vi "MainImage.vi"() -> ()   [LabVIEW 2019]
panel:
  in  "stop":bool
  in  "Tab Control":enum32{"Pressure", "Temperature", "Image"}(tab)
  out "Waveform Chart 2":cluster{dbl, dbl, dbl}(graph)
  in  "VISA resource name":refnum<visa-resource-name>="COM3"
  in  "termination char\n(0xA = '\\n' = LF)":u8=13 format="%.0x"
  in  "Recieve Data":bool
  out "Waveform Chart":T1(graph)
  in  "physical channels":tag="PXI1Slot2/ai2"
  in  "resistance configuration":i32(ring)=2 items=["2-Wire"=2, "3-Wire"=3, "4-Wire"=4]
  in  "valor":i32
  out "Gauge 1":dbl
  out "Gauge 2":dbl
  out "Gauge 3":dbl
  out "Thermometer":dbl(slide) scale=0.0..100.0
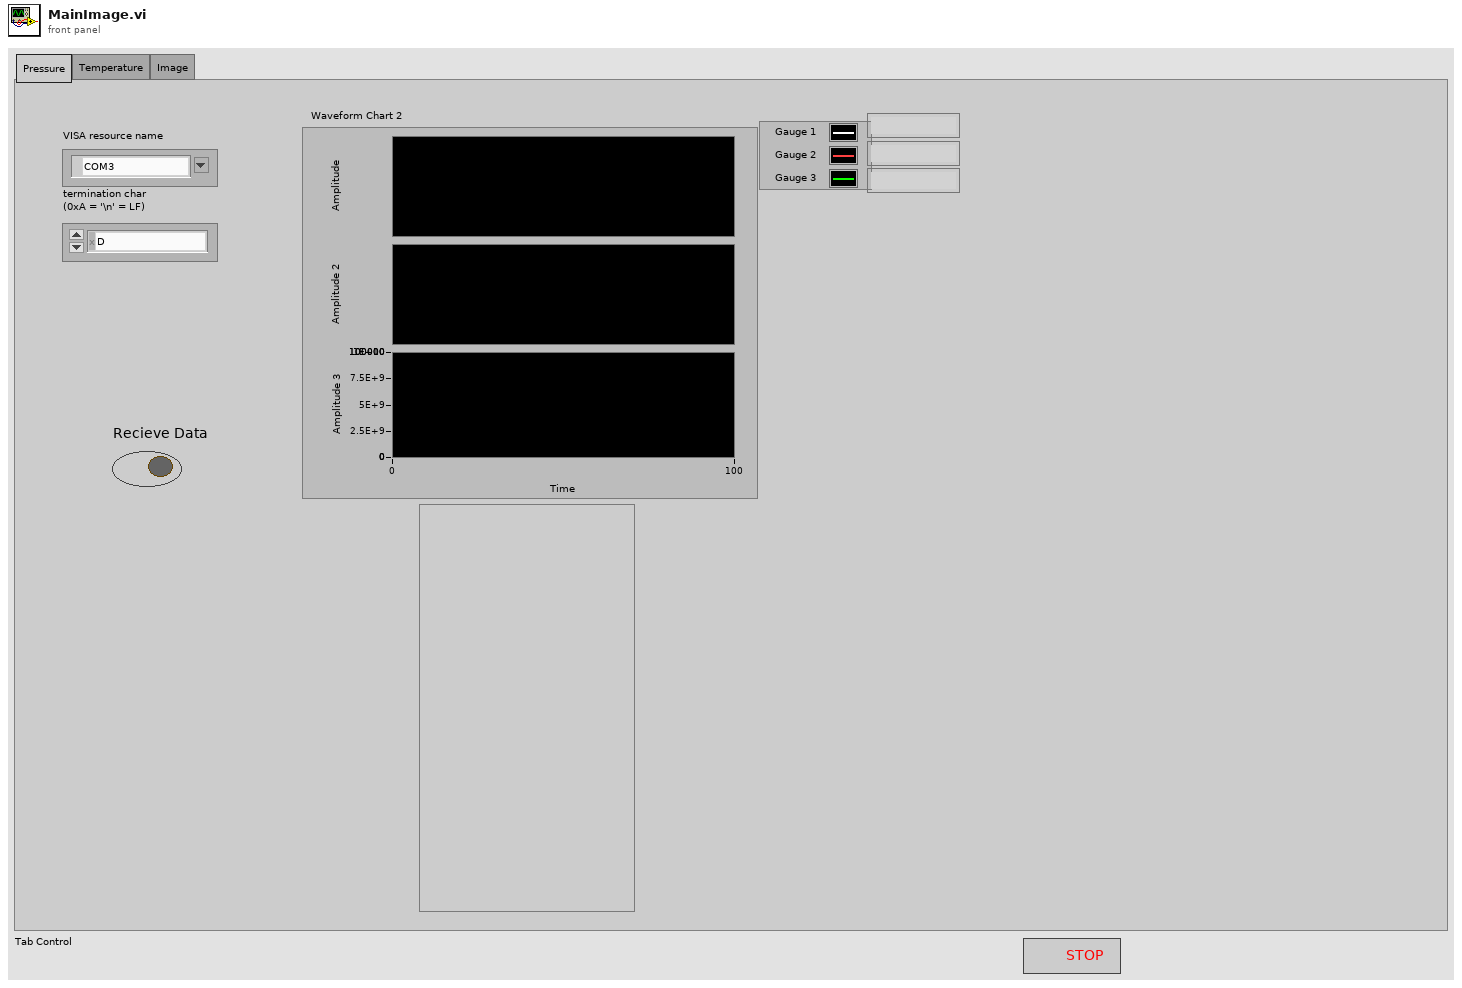
[diagram p1: front panel]
types:
  T1 = cluster{"data[0]":dbl, "data[1]":dbl, "data[2]":dbl, "data[3]":dbl, "data[4]":dbl, "data[5]":dbl, "data[6]":dbl, "data[7]":dbl, "data[8]":dbl, "data[9]":dbl}
  T2 = enum16{"open", "replace", "create", "open or create", "replace or create", "replace or create with confirmation"}
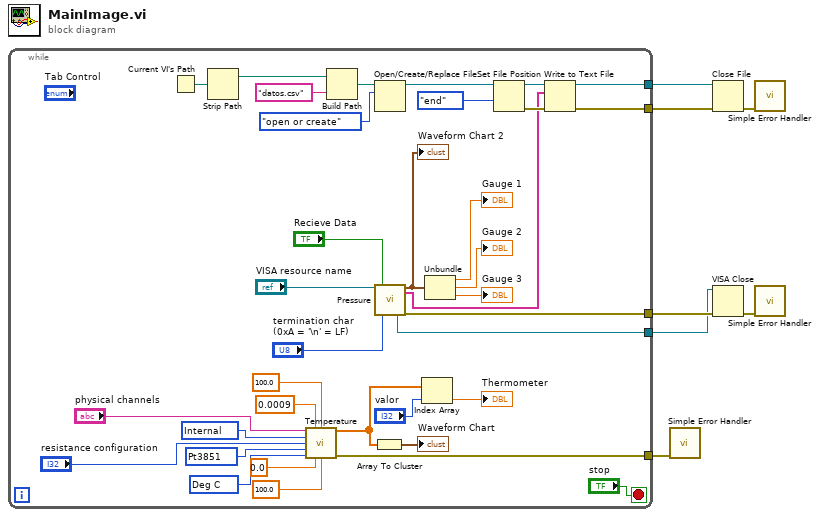
[diagram p0: block diagram]
diagram:
  n1 = while {
    tunnel: [w39] -> w7
    tunnel: [w38] -> w6
    tunnel: [w37] -> w4
    tunnel: [w26] -> w2
    tunnel: [w25] -> w1
    stop <- "stop" stop-if-true
    w16 = 10143 items=["Deg C"=10143, "Deg F"=10144, "Kelvins"=10325, "Deg R"=10145, "From Custom Scale"=10065] ("units")
    w17 = 10071 items=["Pt3750"=12481, "Pt3851"=10071, "Pt3911"=12482, "Pt3916"=10069, "Pt3920"=10053, "Pt3928"=12483, "Custom"=10137] ("rtd type")
    w18 = 10200 items=["Internal"=10200, "External"=10167, "None"=10230] ("current excitation source")
    n2 = Current VI's Path() -> (path=w33:path)
    n3 = Strip Path(path=w33) -> (stripped path=w34:path)  [unwired: 1 out]
    n4 = call "Temperature.vi"("physical channels"="physical channels", "current excitation value"=0.0009, "r0"=100.0, "current excitation source"=w18, "resistance configuration"="resistance configuration", "rtd type"=w17, "units"=w16, "minimum value"=0.0, "maximum value"=100.0) -> ("data"=w21:dbl[], "error out"=w37:errorcluster)  [unwired: 5 in]
    n5 = Build Path(base path=w34, name or relative path="datos.csv") -> (appended path=w35:path)
    n6 = Array To Cluster(array=w21) -> (cluster=→"Waveform Chart":T1)
    n7 = Open/Create/Replace File(file path (use dialog)=w35, operation (0:open)=T2."open or create") -> (refnum out=w36:refnum<file>)  [unwired: 4 in, 2 out]
    n8 = call "Pressure.vi"("VISA resource name"="VISA resource name", "Recieve Data"="Recieve Data", "termination char\n(0xA = '\\n' = LF)"="termination char\n(0xA = '\\n' = LF)") -> ("VISA resource name out"=w38:refnum<visa-resource-name>, "output cluster"=w11:cluster{dbl, dbl, dbl}, "output array"=w27:string[], "error out"=w39:errorcluster)  [unwired: 10 in, 3 out]
    "Waveform Chart 2" <- w11
    n9 = Index Array(array=w21, index="valor") -> (element=→"Thermometer":dbl)
    n10 = Unbundle(w11) -> (→"Gauge 1":dbl, →"Gauge 2":dbl, →"Gauge 3":dbl)
    n11 = Set File Position(refnum=w36, from (0:start)=enum16{"start", "end", "current"}."end") -> (refnum out=w29:refnum<file>, error out=w28:errorcluster)  [unwired: 2 in]
    n12 = Write to Text File(file (use dialog)=w29, text=w27, error in=w28) -> (refnum out=w26:refnum<file>, error out=w25:errorcluster)  [unwired: 1 in, 1 out]
  }
  n13 = call <vilib>:"Simple Error Handler.vi"("error in (no error)"=w4) -> ()  [unwired: 4 in, 5 out]
  n14 = Close File(refnum=w2, error in=w1) -> (error out=w3:errorcluster)  [unwired: 1 out]
  n15 = VISA Close(VISA resource name=w6, error in (no error)=w7) -> (error out=w5:errorcluster)
  n16 = call <vilib>:"Simple Error Handler.vi"("error in (no error)"=w3) -> ()  [unwired: 1 in, 8 out]
  n17 = call <vilib>:"Simple Error Handler.vi"("error in (no error)"=w5) -> ()  [unwired: 4 in, 5 out]
